vi "CAN_Init-donotOpen.vi"(0 "设备类型":u32(ring)=4 items=["PCI5121"=1, "PCI9810"=2, "USBCAN1"=3, "USBCAN2"=4, "PCI9820"=5, "CAN232"=6, "PCI5110"=7, "CANLite(mini)"=8, "ISA9620"=9, "ISA5420"=10, "PC104CAN"=11, "CANET"=17, "DNP9810"=13, "USBCAN-E-U"=20, "USBCAN-2E-U"=21], 1 "设备索引":u32(ring) items=["0", "1", "2", "3", "4", "5", "6", "7", "8", "9", "10", "11", "12", "13", "14", "15", ""], 2 "波特率":enum16{"250Kbps", "500Kbps"}(ring)=enum."500Kbps", 3 "CAN路数":u32(ring) items=["0", "1"], 4 "操作类型":enum16{"初始化CAN", "关闭CAN"}(ring), 5 "error in (no error)":errorcluster caption="错误输入（无错误）", 6 "滤波方式":u8(ring)=1 items=["Dual Filter", "Single Filter"], 7 "Accept Code":u32 format="%08x", 8 "IP":string, 9 "port":u32, 10 "工作方式":u8(ring) items=["Normal", "Listen Only"], 11 "Mask Code":u32=4294967295 format="%08x", 12 "PC端-协议类型":enum16{"TCP服务器Server", "TCP客户端Client"}(ring)) -> (14 "CAN 操作结果":bool=TRUE, 19 "error out":errorcluster caption="错误输出")   [LabVIEW 2013]
uses:
  data/ControlCAN.dll
panel:
  in  "VCI_INIT_CONFIG":T1={"AccCode"=0, "AccMask"=4294967295, "Reserved"=0, "Filter"=0, "Timing0"=191, "Timing1"=255, "Mode"=0}
  in  "DeviceType 5":u16(ring)=1 items=["PCI5121"=1, "PCI9810"=2, "USBCAN1"=3, "USBCAN2"=4, "PCI9820"=5, "CAN232"=6, "PCI5110"=7, "CANLite(mini)"=8, "ISA9620"=9, "ISA5420"=10, "PC104CAN"=11, "CANETE"=12, "DNP9810"=13]
  in  "CAN Channel 3":u16(ring) items=["0", "1"]
  in  "DeviceType 4":u16(ring)=1 items=["PCI5121"=1, "PCI9810"=2, "USBCAN1"=3, "USBCAN2"=4, "PCI9820"=5, "CAN232"=6, "PCI5110"=7, "CANLite(mini)"=8, "ISA9620"=9, "ISA5420"=10, "PC104CAN"=11, "CANETE"=12, "DNP9810"=13]
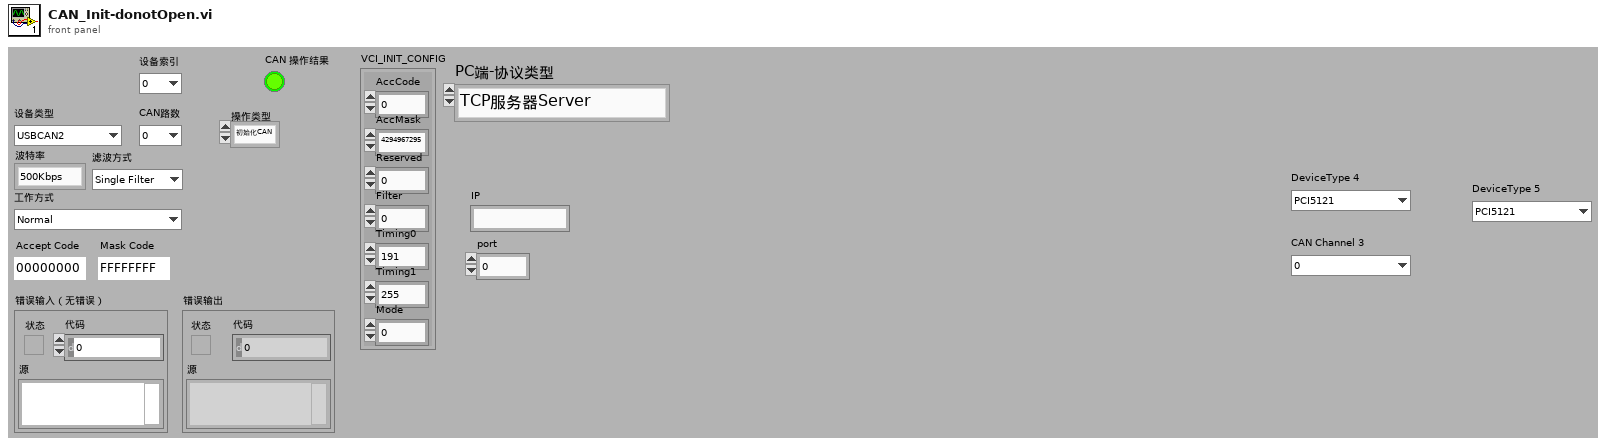
[diagram p1: front panel]
types:
  T1 = cluster{"AccCode":u32, "AccMask":u32, "Reserved":u32, "Filter":u8, "Timing0":u8, "Timing1":u8, "Mode":u8}
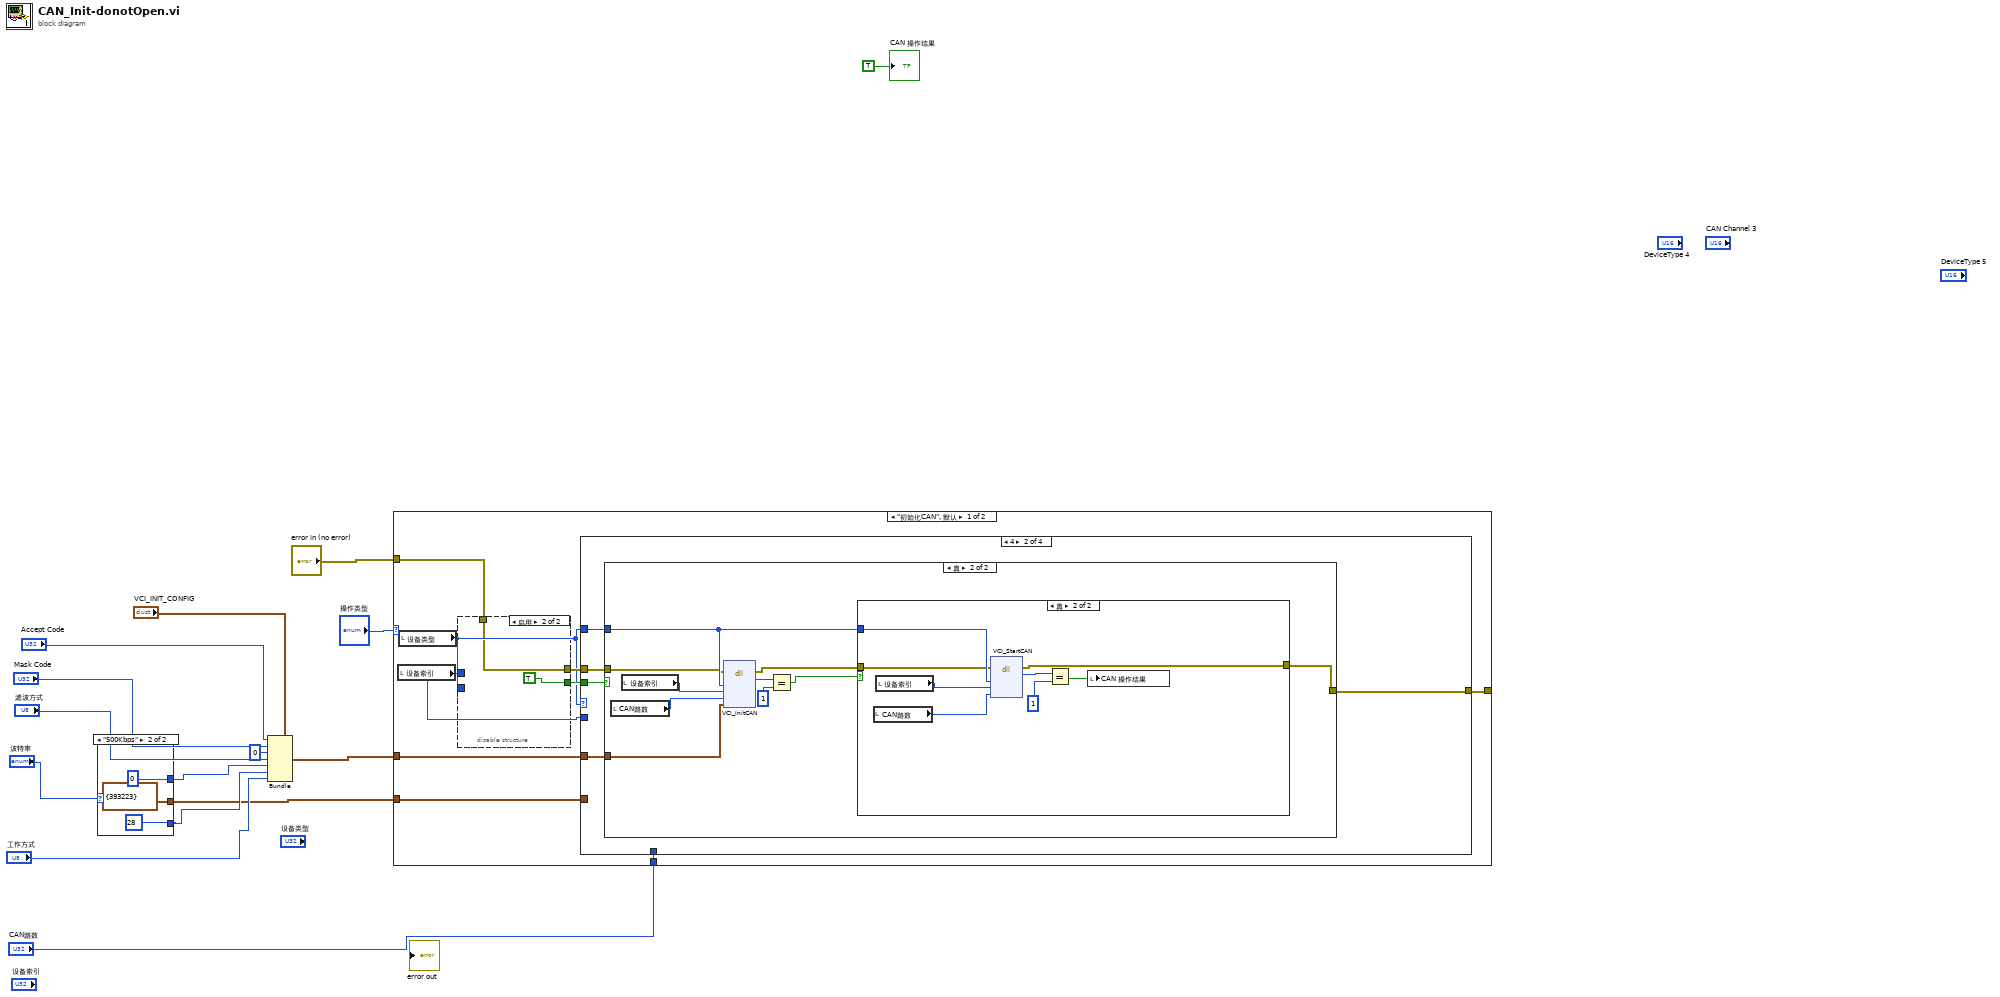
[diagram p0: block diagram]
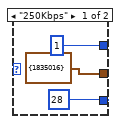
[diagram p2: hidden frame]
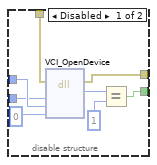
[diagram p3: hidden frame]
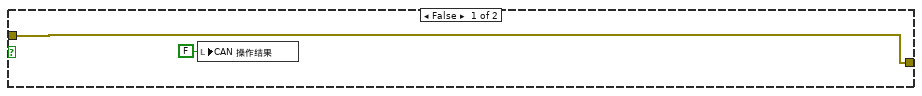
[diagram p5: hidden frame]
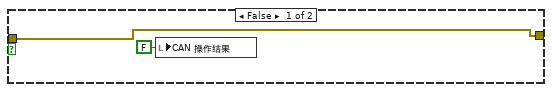
[diagram p6: hidden frame]
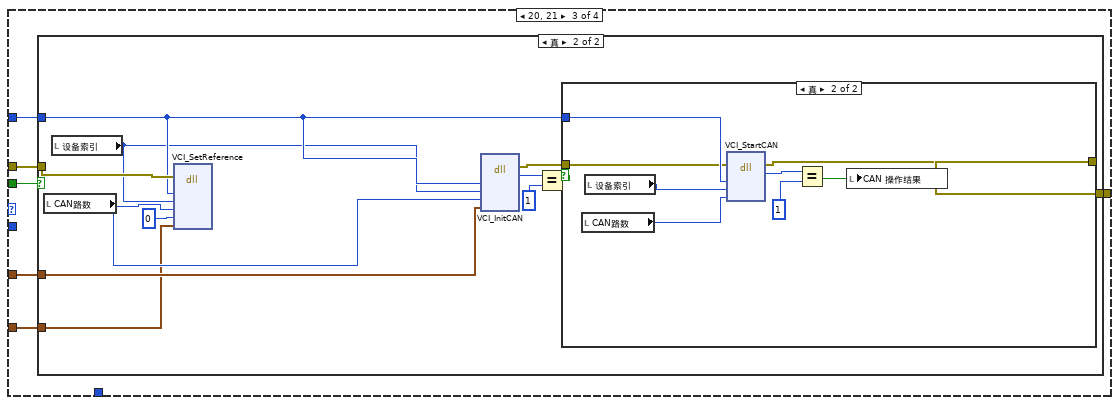
[diagram p7: hidden frame]
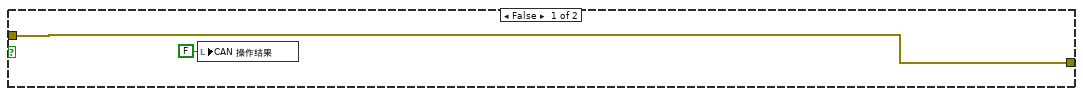
[diagram p8: hidden frame]
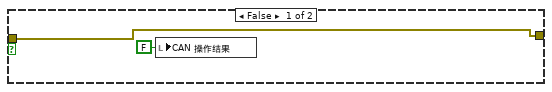
[diagram p9: hidden frame]
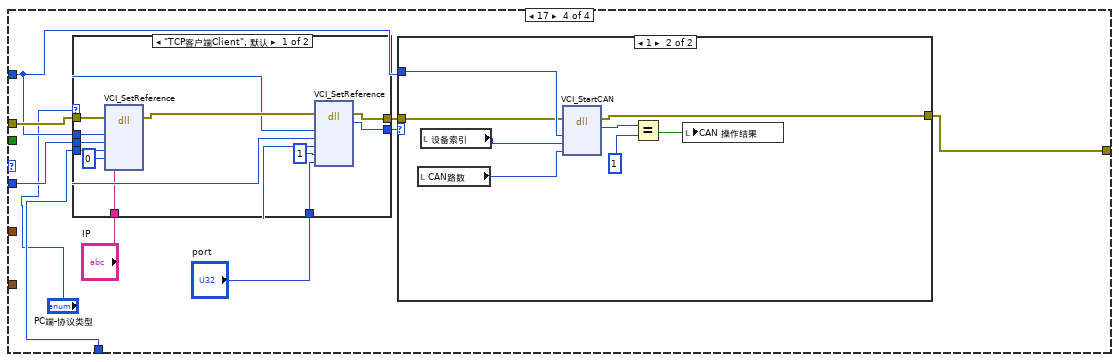
[diagram p10: hidden frame]
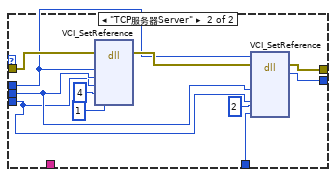
[diagram p11: hidden frame]
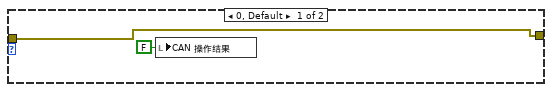
[diagram p12: hidden frame]
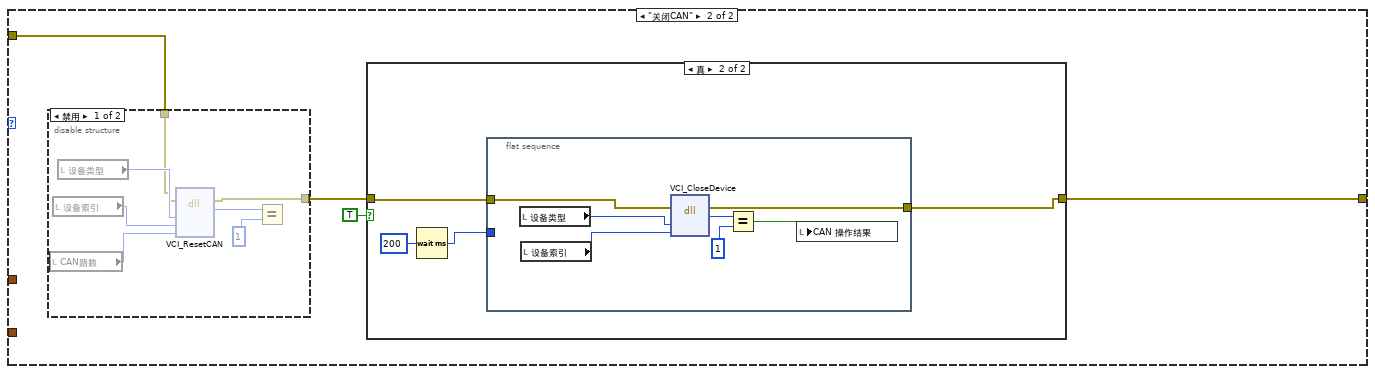
[diagram p13: hidden frame]
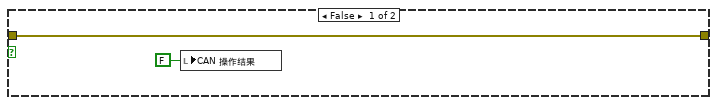
[diagram p15: hidden frame]
diagram:
  n1 = case shown="\"500Kbps\"" "波特率" {
    tunnel: [1 0] -> w14
    tunnel: [28 28] -> w13
    tunnel: [cluster{u32} {1835016} cluster{u32} {393223}] -> w1
    frame "250Kbps" {
    }
    frame "500Kbps" {
    }
  }
  n2 = Bundle(cluster="VCI_INIT_CONFIG", "AccCode"="Accept Code", "AccMask"="Mask Code", "Reserved"=u32 0, "Filter"="滤波方式", "Timing0"=w14, "Timing1"=w13, "Mode"="工作方式") -> (w9:T1)
  n3 = case shown="\"初始化CAN\", 默认" "操作类型" {
    tunnel: w9 -> [w30 _]
    tunnel: "error in (no error)" -> [w29 w144]
    tunnel: [w27 w142] -> _
    tunnel: "CAN路数" -> [w24 _]
    tunnel: w1 -> [w22 _]
    frame "初始化CAN", Default {
      n4 = local read "设备索引"() -> (w25:u32)
      n5 = local read "设备类型"() -> (w23:u32)
      n6 = disable-structure shown="启用" {
        disable-tunnel: w29 -> [w35 w39]
        disable-tunnel: [w34 w39] -> w28
        disable-tunnel: [w33 TRUE] -> w26
        disable-tunnel: w25 -> [w32 _]
        disable-tunnel: w23 -> [w31 _]
        frame Disabled {
          n7 = dll-call lib="PTH1tabs FBluewave New EnergySVN_WorkBMS_Monitor_Bnet01trunkBMS_Monitor_增加二维码dataControlCAN.dll" fn="VCI_OpenDevice"(error in=w35, "DevType"=w31, "DevIndex"=w32, "Reserved"=0) -> (error out=w34:errorcluster, "返回类型"=w37:u32)  [unwired: 3 in, 3 out]
          n8 = Equal?(x=w37, y=u32 1) -> (x = y?=w33:bool)
        }
        frame Enabled {
        }
      }
      n9 = case shown="4" w23 {
        tunnel: w26 -> [_ w46 w74 _]
        tunnel: w23 -> [_ w45 w73 w103]
        tunnel: w30 -> [_ w44 w72 _]
        tunnel: w28 -> [w41 w43 w71 w108]
        tunnel: [w41 w42 w70 w102] -> w27
        tunnel: w25 -> [_ _ _ w107]
        tunnel: w24 -> [_ _ _ w106]
        tunnel: w22 -> [_ _ w69 _]
        frame 0, Default {
        }
        frame 4 {
          n10 = case shown="真" w46 {
            tunnel: w45 -> [_ w53]
            tunnel: w44 -> [_ w52]
            tunnel: w43 -> [w47 w51]
            tunnel: [w47 w49] -> w42
            frame False {
              n11 = local write "CAN 操作结果"(FALSE ("初始化结果")) -> ()
            }
            frame True {
              n12 = local read "CAN路数"() -> (w55:u32)
              n13 = local read "设备索引"() -> (w56:u32)
              n14 = dll-call lib="PTH1tabs FBluewave New EnergySVN_WorkBMS_Monitor_Bnet01trunkBMS_Monitor_增加二维码dataControlCAN.dll" fn="VCI_InitCAN"(error in=w51, "DeviceType"=w53, "DeviceInd"=w56, "CANInd"=w55, "pInitConfig"=w52) -> (error out=w50:errorcluster, "返回类型"=w57:u32)  [unwired: 3 in, 4 out]
              n15 = Equal?(x=w57, y=u32 1) -> (x = y?=w54:bool)
              n16 = case shown="真" w54 {
                tunnel: w53 -> [_ w66]
                tunnel: w50 -> [w59 w62]
                tunnel: [w59 w61] -> w49
                frame False {
                  n17 = local write "CAN 操作结果"(FALSE ("初始化结果")) -> ()
                }
                frame True {
                  n18 = local read "CAN路数"() -> (w64:u32)
                  n19 = local read "设备索引"() -> (w65:u32)
                  n20 = dll-call lib="PTH1tabs FBluewave New EnergySVN_WorkBMS_Monitor_Bnet01trunkBMS_Monitor_增加二维码dataControlCAN.dll" fn="VCI_StartCAN"(error in=w62, "DeviceType"=w66, "DeviceInd"=w65, "CANInd"=w64) -> (error out=w61:errorcluster, "返回类型"=w67:u32)  [unwired: 2 in, 4 out]
                  n21 = Equal?(x=w67, y=u32 1) -> (x = y?=w63:bool)
                  n22 = local write "CAN 操作结果"(w63) -> ()
                }
              }
            }
          }
        }
        frame 20, 21 {
          n23 = case shown="真" w74 {
            tunnel: w73 -> [_ w80]
            tunnel: w72 -> [_ w85]
            tunnel: w71 -> [w75 w82]
            tunnel: [w75 w83] -> w70
            tunnel: w69 -> [_ w77]
            frame False {
              n24 = local write "CAN 操作结果"(FALSE ("初始化结果")) -> ()
            }
            frame True {
              n25 = local read "CAN路数"() -> (w78:u32)
              n26 = local read "设备索引"() -> (w79:u32)
              n27 = dll-call lib="PTH1tabs FBluewave New EnergySVN_WorkBMS_Monitor_Bnet01trunkBMS_Monitor_增加二维码dataControlCAN.dll" fn="VCI_SetReference" label="VCI_SETREF"(error in=w82, "DeviceType"=w80, "DeviceInd"=w79, "CANInd"=w78, "RefType"=u32 0, "pData"=w77) -> ()  [unwired: 4 in, 6 out]
              n28 = dll-call lib="PTH1tabs FBluewave New EnergySVN_WorkBMS_Monitor_Bnet01trunkBMS_Monitor_增加二维码dataControlCAN.dll" fn="VCI_InitCAN"("DeviceType"=w80, "DeviceInd"=w79, "CANInd"=w78, "pInitConfig"=w85) -> (error out=w84:errorcluster, "返回类型"=w87:u32)  [unwired: 4 in, 4 out]
              n29 = Equal?(x=w87, y=u32 1) -> (x = y?=w86:bool)
              n30 = case shown="真" w86 {
                tunnel: w80 -> [_ w96]
                tunnel: w84 -> [w89 w92]
                tunnel: [w89 w91] -> w83
                frame False {
                  n31 = local write "CAN 操作结果"(FALSE ("初始化结果")) -> ()
                }
                frame True {
                  n32 = local read "CAN路数"() -> (w94:u32)
                  n33 = local read "设备索引"() -> (w95:u32)
                  n34 = dll-call lib="PTH1tabs FBluewave New EnergySVN_WorkBMS_Monitor_Bnet01trunkBMS_Monitor_增加二维码dataControlCAN.dll" fn="VCI_StartCAN"(error in=w92, "DeviceType"=w96, "DeviceInd"=w95, "CANInd"=w94) -> (error out=w91:errorcluster, "返回类型"=w97:u32)  [unwired: 2 in, 4 out]
                  n35 = Equal?(x=w97, y=u32 1) -> (x = y?=w93:bool)
                  n36 = local write "CAN 操作结果"(w93) -> ()
                }
              }
            }
          }
        }
        frame 17 {
          n37 = case shown="\"TCP客户端Client\", 默认" "PC端-协议类型" {
            tunnel: w108 -> [w119 w125]
            tunnel: w107 -> [w116 w122]
            tunnel: w106 -> [w115 w121]
            tunnel: [w113 w129] -> w105
            tunnel: [w112 w128] -> w104
            tunnel: w103 -> [w111 w123]
            tunnel: "IP" -> [w110 _]
            tunnel: "port" -> [w109 w127]
            frame "TCP客户端Client", Default {
              n38 = dll-call lib="PTH1tabs FBluewave New EnergySVN_WorkBMS_Monitor_Bnet01trunkBMS_Monitor_增加二维码dataControlCAN.dll" fn="VCI_SetReference" label="VCI_SETREF"(error in=w119, "DeviceType"=w111, "DeviceInd"=w116, "CANInd"=w115, "RefType"=u32 0, "pData"=w110) -> (error out=w117:errorcluster)  [unwired: 4 in, 5 out]
              n39 = dll-call lib="PTH1tabs FBluewave New EnergySVN_WorkBMS_Monitor_Bnet01trunkBMS_Monitor_增加二维码dataControlCAN.dll" fn="VCI_SetReference" label="VCI_SETREF"(error in=w117, "DeviceType"=w111, "DeviceInd"=w116, "CANInd"=w115, "RefType"=u32 1, "pData"=w109) -> (error out=w113:errorcluster, "返回类型"=w112:u32)  [unwired: 4 in, 4 out]
            }
            frame "TCP服务器Server" {
              n40 = dll-call lib="PTH1tabs FBluewave New EnergySVN_WorkBMS_Monitor_Bnet01trunkBMS_Monitor_增加二维码dataControlCAN.dll" fn="VCI_SetReference" label="VCI_SETREF"(error in=w125, "DeviceType"=w123, "DeviceInd"=w122, "CANInd"=w121, "RefType"=u32 4, "pData"=u32 1) -> (error out=w124:errorcluster)  [unwired: 4 in, 5 out]
              n41 = dll-call lib="PTH1tabs FBluewave New EnergySVN_WorkBMS_Monitor_Bnet01trunkBMS_Monitor_增加二维码dataControlCAN.dll" fn="VCI_SetReference" label="VCI_SETREF"(error in=w124, "DeviceType"=w123, "DeviceInd"=w122, "CANInd"=w121, "RefType"=u32 2, "pData"=w127) -> (error out=w129:errorcluster, "返回类型"=w128:u32)  [unwired: 4 in, 4 out]
            }
          }
          n42 = case shown="1" w104 {
            tunnel: w103 -> [_ w138]
            tunnel: w105 -> [w131 w134]
            tunnel: [w131 w133] -> w102
            frame 0, Default {
              n43 = local write "CAN 操作结果"(FALSE ("初始化结果")) -> ()
            }
            frame 1 {
              n44 = local read "CAN路数"() -> (w136:u32)
              n45 = local read "设备索引"() -> (w137:u32)
              n46 = dll-call lib="PTH1tabs FBluewave New EnergySVN_WorkBMS_Monitor_Bnet01trunkBMS_Monitor_增加二维码dataControlCAN.dll" fn="VCI_StartCAN"(error in=w134, "DeviceType"=w138, "DeviceInd"=w137, "CANInd"=w136) -> (error out=w133:errorcluster, "返回类型"=w139:u32)  [unwired: 2 in, 4 out]
              n47 = Equal?(x=w139, y=u32 1) -> (x = y?=w135:bool)
              n48 = local write "CAN 操作结果"(w135) -> ()
            }
          }
        }
      }
    }
    frame "关闭CAN" {
      n49 = disable-structure shown="禁用" {
        disable-tunnel: w144 -> [w146 w152]
        disable-tunnel: [w145 w152] -> w143
        frame Disabled {
          n50 = local read "CAN路数"() -> (w147:u32)
          n51 = local read "设备索引"() -> (w148:u32)
          n52 = local read "设备类型"() -> (w149:u32)
          n53 = dll-call lib="PTH1tabs FBluewave New EnergySVN_WorkBMS_Monitor_Bnet01trunkBMS_Monitor_增加二维码dataControlCAN.dll" fn="VCI_ResetCAN"(error in=w146, "DeviceType"=w149, "DeviceInd"=w148, "CANInd"=w147) -> (error out=w145:errorcluster, "返回类型"=w150:u32)  [unwired: 2 in, 4 out]
          n54 = Equal?(x=w150, y=u32 1) -> ()  [unwired: 1 out]
        }
        frame Enabled {
        }
      }
      n55 = case shown="真" TRUE {
        tunnel: w143 -> [w153 w158]
        tunnel: [w153 w157] -> w142
        frame False {
          n56 = local write "CAN 操作结果"(FALSE ("CAN 操作结果")) -> ()
        }
        frame True {
          n57 = Wait (ms)(milliseconds to wait=u32 200 ("等待时间（毫秒）")) -> (millisecond timer value=w155:u32)
          n58 = flat-sequence {
            tunnel: w158 -> [w160]
            tunnel: [w159] -> w157
            tunnel: w155 -> [_]
            frame #0 {
              n59 = local read "设备类型"() -> (w163:u32)
              n60 = local read "设备索引"() -> (w162:u32)
              n61 = dll-call lib="PTH1tabs FBluewave New EnergySVN_WorkBMS_Monitor_Bnet01trunkBMS_Monitor_增加二维码dataControlCAN.dll" fn="VCI_CloseDevice"(error in=w160, "DeviceType"=w163, "DeviceInd"=w162) -> (error out=w159:errorcluster, "返回类型"=w164:u32)  [unwired: 2 in, 3 out]
              n62 = Equal?(x=w164, y=u32 1) -> (x = y?=w161:bool)
              n63 = local write "CAN 操作结果"(w161) -> ()
            }
          }
        }
      }
    }
  }
  "CAN 操作结果" <- TRUE ("CAN 操作结果")
